vi "Copy Library.vi"(8 "error in":errorcluster, 11 "library":refnum<vi>) -> (0 "error out":errorcluster, 2 "New Library Path":path, 3 "library out":refnum<vi>)   [LabVIEW 2024, in "gRPC Client Generation.lvlib"]
uses:
  gRPC Client Generation.lvlib
  7ec7ef9e-7412-4a39-8ea6-48729f3c173f.vi
  <vilib>/Comparison/Equal/Equal Functor/Equal Functor.lvclass
panel:
  out "resulting string":string
  out "lowercase file extension":string
  out "stripped path":path
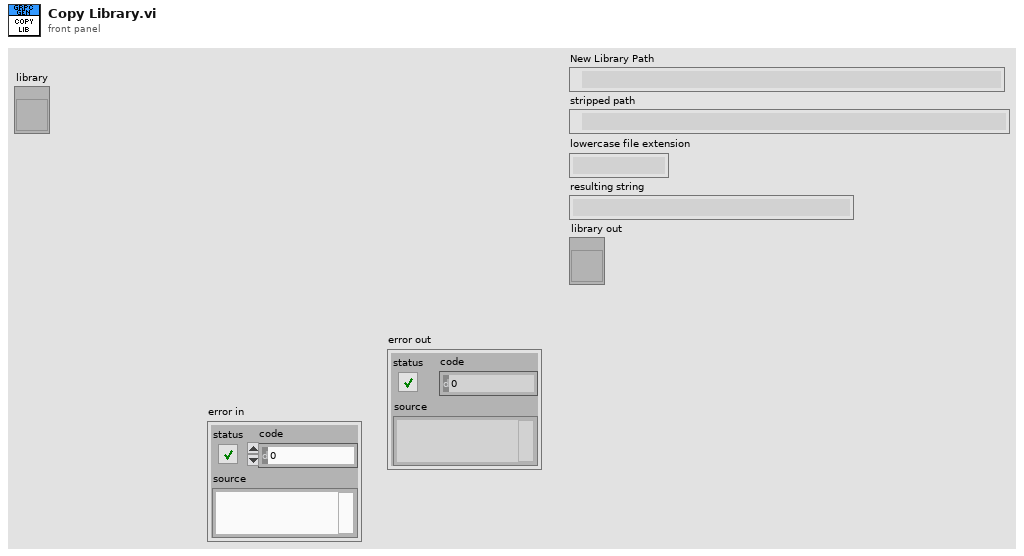
[diagram p1: front panel]
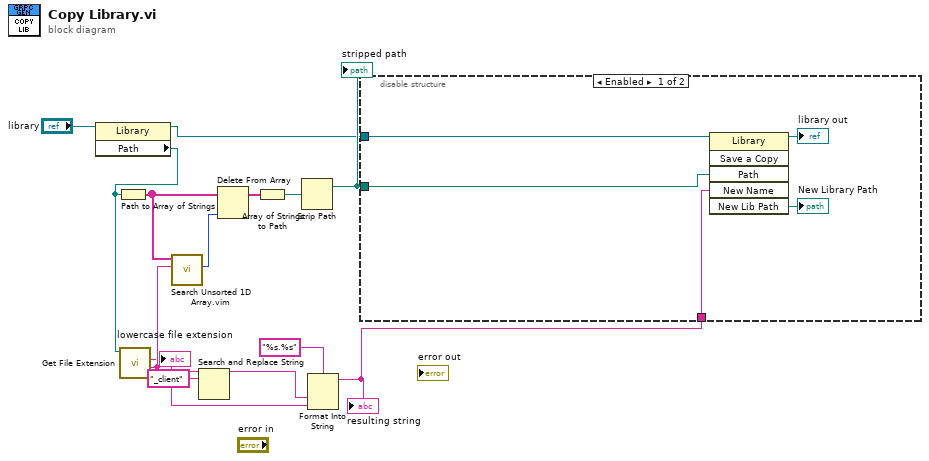
[diagram p0: block diagram]
diagram:
  n1 = property class="Library"(reference="library") -> (reference out=w1:refnum<vi>, "Path"=w12:path)  [unwired: 1 in, 1 out]
  n2 = Path to Array of Strings(0:w12) -> (2:w11:string[])  [unwired: 1 out]
  n3 = call <vilib>:"Get File Extension.vi"("file"=w12) -> ("filename without extension"=w8:string, "lowercase file extension"=w4:string)  [unwired: 6 in, 3 out]
  "lowercase file extension" <- w4
  n4 = call "Search Unsorted 1D Array.vim"("element"=w8, "unsorted 1D array"=w11) -> ("index of element"=w13:i32)  [unwired: 9 in]
  n5 = Search and Replace String(input string=w8, search string="_client") -> (result string=w5:string)  [unwired: 6 in, 3 out]
  n6 = Delete From Array(array=w11, index=w13) -> (array with subset deleted=w10:string[])  [unwired: 1 in, 1 out]
  n7 = Array of Strings to Path(0:w10) -> (2:w9:path)  [unwired: 1 in]
  n8 = Strip Path(path=w9) -> (stripped path=w3:path)  [unwired: 1 out]
  "stripped path" <- w3
  n9 = Format Into String(format string="%s.%s", w5, w4) -> (resulting string=w2:string)  [unwired: 2 in, 1 out]
  "resulting string" <- w2
  n10 = disable-structure shown="Enabled" {
    disable-tunnel: w3 -> [w18 _]
    disable-tunnel: w2 -> [w17 _]
    disable-tunnel: w1 -> [w16 _]
    frame Enabled {
      n11 = invoke class="Library" method="Save a Copy"(reference=w16, "Path"=w18, "New Name"=w17) -> (reference out=→"library out":refnum<vi>, "New Lib Path"=→"New Library Path":path)  [unwired: 3 in, 4 out]
    }
    frame Disabled {
    }
  }
